vi "Basic Serial Write and Read.vi"(0 "VISA resource name":refnum<visa-resource-name>="COM1", 1 "baud rate":u32=9600, 2 "data bits":u16=8 min=5 max=8 step=1, 3 "parity":u16(ring) items=["None", "Odd", "Even", "Mark", "Space"], 4 "stop bits":u16(ring)=10 items=["1.0"=10, "1.5"=15, "2.0"=20], 5 "write":bool=TRUE, 6 "read":bool=TRUE, 7 "flow control":u16(ring) items=["None"=0, "XON/XOFF"=1, "RTS/CTS"=2, "DTR/DSR"=4], 8 "string to write":string="*IDN?\n") -> (9 "read string":string, 10 "bytes read":u32)   [LabVIEW 2011]
doc: "The Basic Serial Read and Write example performs a Serial Port Read, a Serial Port Write, or a combination of these actions. The user selects the actions (read or write) on the front panel. If both are selected, the VI will write the data first, read data, and then close the VISA session that is opened to the port. This VI will wait until the specified number of bytes is received at the port or until a termination character is read.\n\nINSTRUCTIONS:\n1) Select the serial resource and configuration parameters (baud rate, data bits, parity, stop bits, flow control).\n2) Select the operations to be performed. \n3) Connect the serial port to your device. If no device is available, perform a loopback test by doing one of the following. Short pins 2 and 3 on a RS-232 cable or short pin 4 to pin 8 and pin 5 to pin 9 on a RS-485/422 cable. \n4) Run the VI to see the data read. (The \"read string\" will match the \"string to write\" if a loopback test was performed.)\n\nNote: The parameters set for the serial port must match the parameters of the connected instrument or device. In this example, the bytes to read parameter specifies the number of bytes that the serial port reads. If there were more bytes at the port than the number specified in bytes to read, those bytes would not be read. Also, if you specify to read more bytes than the number of bytes actually read, you might receive a timeout error message.\n\nOn the block diagram, the Configure Serial Port VI sets the configuration parameters. The front panel displays the controls used to configure the basic parameters, such as baud rate, data bits, and parity. Constants configure the other parameters the user probably does not need set. After the VISA Configure Serial Port VI opens the VISA session and configures the port, the VI passes the VISA resource name to other VIs that perform operations on that VISA resource. The VISA Write function sends a command to the serial device and the VISA Read function returns data based on the command. The VISA Close function then closes the reference to the serial device. It is important to close the reference; otherwise communication through with that port through protocols other than VISA might not be possible."
uses:
  <vilib>/Instr/_visa.llb/VISA Configure Serial Port (Instr).vi
panel:
  in  "delay before read (ms)":u32=500
  # "On Windows/Linux, consider using the Instrument Driver Finder (Help>>Find Instrument Drivers) to search for an instrument driver for your instrument."
  # "Select the serial resource and the operations (Read, Write, or both) to be performed.  If both are selected, the VI will write the data first, read data and then close the VISA session that is opened to the port.  This VI will wait until the specified number of bytes is received at the port or until a termination character is read."
  # "For additional information select File >> VI Properties >> Documentation"
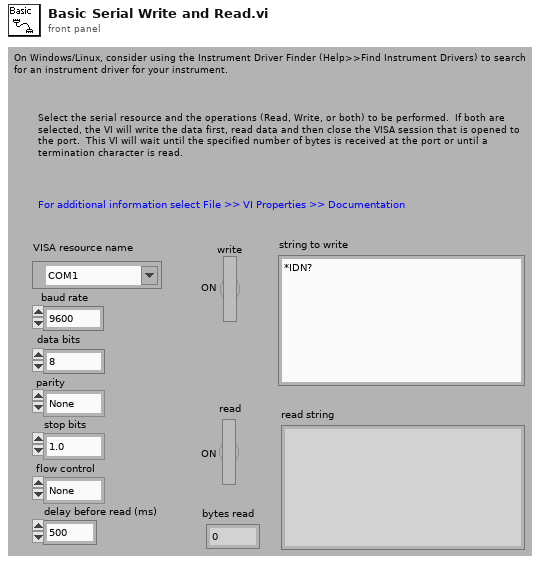
[diagram p1: front panel]
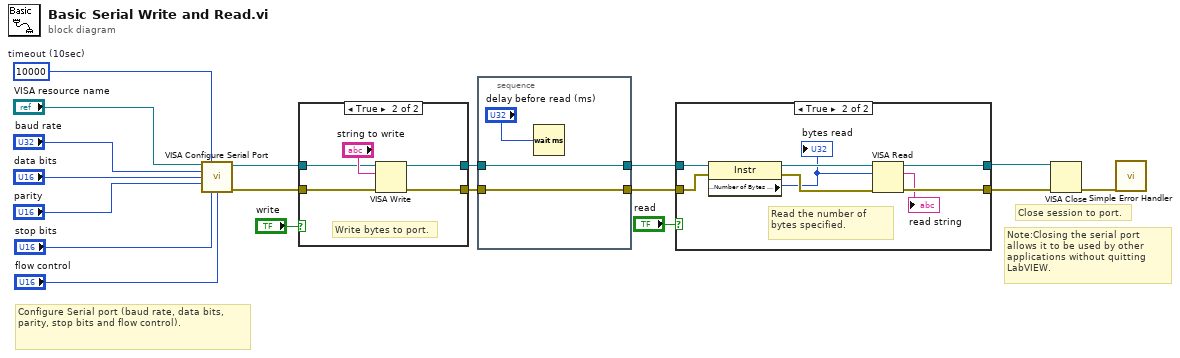
[diagram p0: block diagram]
diagram:
  w9 = u32 10000  # timeout (10sec)
  # "Note:Closing the serial port allows it to be used by other applications without quitting LabVIEW."
  # "Configure Serial port (baud rate, data bits, parity, stop bits and flow control)."
  # "Close session to port."
  n1 = call-poly "VISA Configure Serial Port"("VISA resource name"="VISA resource name", "timeout (10sec)"=w9, "baud rate (9600)"="baud rate", "data bits (8)"="data bits", "parity (0:none)"="parity", "stop bits (10: 1 bit)"="stop bits", "flow control (0:none)"="flow control") -> ("VISA resource name out"=w14:refnum<visa-resource-name>, "error out"=w15:errorcluster)  [unwired: 1 in, 6 out]
  n2 = case shown="True" "write" {
    tunnel: [w20 w25] -> w4
    tunnel: w14 -> [w19 w23]
    tunnel: w15 -> [w20 w22]
    tunnel: [w19 w21] -> w2
    frame False {
    }
    frame True {
      # "Write bytes to port."
      n3 = VISA Write(VISA resource name=w23, write buffer="string to write", error in (no error)=w22) -> (VISA resource name out=w21:refnum<visa-resource-name>, error out=w25:errorcluster)  [unwired: 1 out]
    }
  }
  n4 = stacked-sequence {
    tunnel: w4 -> [w28]
    tunnel: [w28] -> w3
    tunnel: w2 -> [w27]
    tunnel: [w27] -> w1
    frame #0 {
      n5 = Wait (ms)(milliseconds to wait="delay before read (ms)") -> ()  [unwired: 1 out]
    }
  }
  n6 = case shown="True" "read" {
    tunnel: w3 -> [w30 w34]
    tunnel: [w30 w38] -> w13
    tunnel: [w29 w37] -> w12
    tunnel: w1 -> [w29 w36]
    frame False {
    }
    frame True {
      # "Read the number of bytes specified."
      n7 = property class="Instr"(reference=w36, error in=w34) -> (reference out=w35:refnum<visa-resource-name>, error out=w33:errorcluster, "Serial Settings:Number of Bytes at Serial Port"=w31:u32)
      "bytes read" <- w31
      n8 = VISA Read(VISA resource name=w35, byte count=w31, error in (no error)=w33) -> (VISA resource name out=w37:refnum<visa-resource-name>, read buffer=→"read string":string, error out=w38:errorcluster)  [unwired: 1 out]
    }
  }
  n9 = VISA Close(VISA resource name=w12, error in (no error)=w13) -> (error out=w11:errorcluster)
  n10 = call <vilib>:"Simple Error Handler.vi"("error in (no error)"=w11) -> ()  [unwired: 1 in, 8 out]
